vi "Read Device ID Type Request.vi"(8 "error in":errorcluster, 9 "Object ID":u8, 10 "Read Device ID Code":T1) -> (0 "error out":errorcluster, 2 "modbus data unit out":refnum<class "Modbus Data Unit.lvclass">)   [LabVIEW 2021, in "Master Function Definition.lvclass"]
doc: "This VI forms the modbus data unit for reading the device identification."
uses:
  Master Function Definition.lvclass
  Modbus Data Unit/Modbus Data Unit.lvclass
  Read Device ID code.ctl
  Modbus Data Unit/Function.ctl
  Modbus Data Unit/Modbus Data Unit.lvclass/Modbus Data Unit.ctl
  Modbus Data Unit/Construct PDU.vi
  Master Function Definition.lvclass/Master Function Definition.ctl
  Data Model/Device Data Model.lvclass
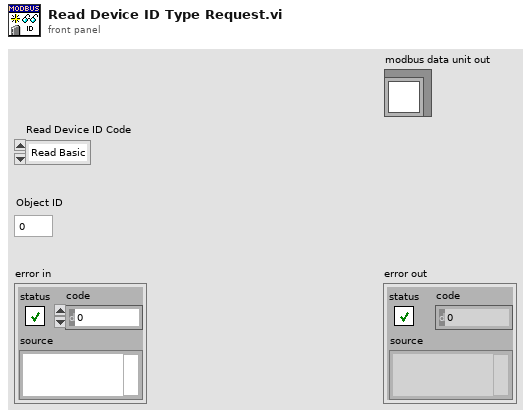
[diagram p1: front panel]
types:
  T1 = typedef "Device Data Model.lvclass/Read Device ID code.ctl" = enum8{"Read Basic", "Read Regular", "Read Extended", "Read Specific"}
  T2 = typedef "Modbus Data Unit.lvclass/Function.ctl" = u8
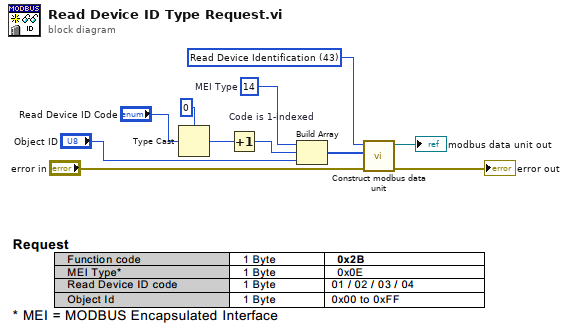
[diagram p0: block diagram]
diagram:
  w6 = u8 14  # MEI Type
  w7 = T2 43 items=["Read Discrete Inputs"=2, "Read Coils"=1, "Write Single Coil"=5, "Write Multiple Coils"=15, "Read Input Register"=4, "Read Holding Registers"=3, "Write Single Register"=6, "Write Multiple Registers"=16, "Read/Write Multiple Registers"=23, "Mask Write Register"=22, "Read FIFO Queue"=24, "Read File Record"=20, "Write File Record"=21, "Read Exception Status"=7, "Diagnostic"=8, "Get Com Event Counter"=11, "Get Com Event Log"=12, "Report Slave ID"=17, "Read Device Identification"=43] ("Function")
  n1 = Type Cast(type=u8 0 ("MEI Type 2"), x="Read Device ID Code") -> (*(type *) &x=w3:u8)
  n2 = Increment "Code is 1-indexed"(x=w3) -> (x+1=w1:u8)
  n3 = Build Array(w6, w1, "Object ID") -> (w8:u8[])
  n4 = call "Construct modbus data unit.vi"("error in"="error in", "data"=w8, "Function"=w7) -> ("error out"=→"error out":errorcluster, "modbus data unit out"=→"modbus data unit out":refnum<class "Modbus Data Unit.lvclass">)  [unwired: 7 in]
